vi "Acquire and process.vi"(7 "Rectangle":T2, 8 "error in (no error)":errorcluster, 9 "Substract images?":bool=TRUE, 10 "Image array":T1[](array[typedef]), 11 "Cam session":T3) -> (0 "error out":errorcluster, 2 "Trimmed image":T1, 3 "Mean Value":sgl)   [LabVIEW 2020]
doc: "Obtains the mean value a ROI maked by Rectangle. Is Substract images? is set toTrue, a difference is calculated between the base image and a newly acquired image before calculating the mean value."
uses:
  <vilib>/userdefined/High Color/IMAQdx.ctl
  <vilib>/vision/Image Controls.llb/IMAQ Image.ctl
  <vilib>/vision/driver/NI_Vision_Acquisition_Software.lvlib
  <vilib>/vision/NI_Vision_Development_Module.lvlib
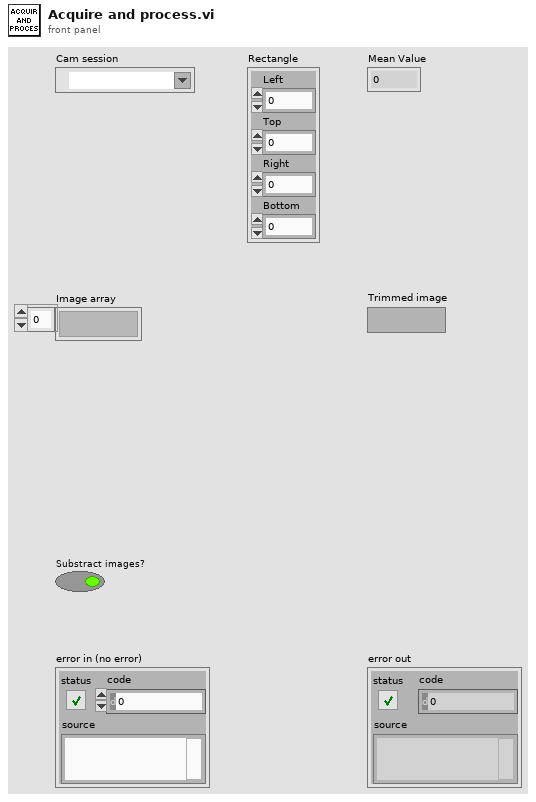
[diagram p1: front panel]
types:
  T1 = typedef "IMAQ Image.ctl" = refnum<image>
  T2 = cluster{"Left":i32, "Top":i32, "Right":i32, "Bottom":i32}
  T3 = typedef "IMAQdx.ctl" = refnum<k21>
  T4 = cluster{"Mean Value":sgl, "Standard Variation":sgl, "Minimal Value":sgl, "Maximal Value":sgl, "Area (calibrated)":sgl, "Area (pixels)":i32, "%":sgl}
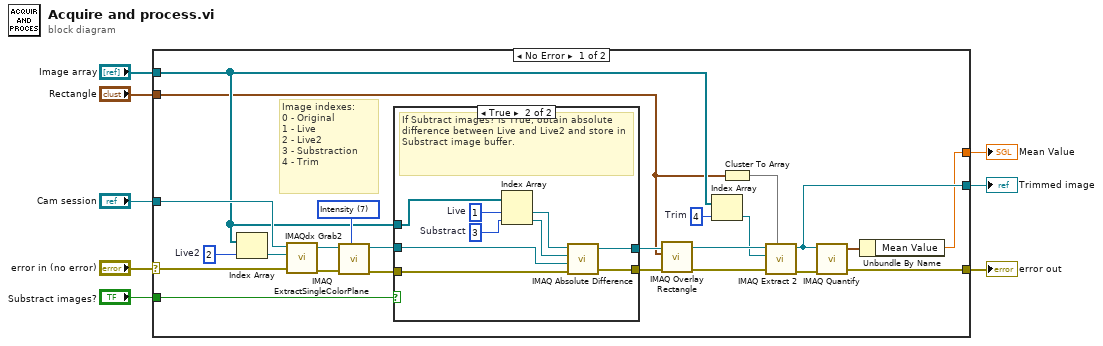
[diagram p0: block diagram]
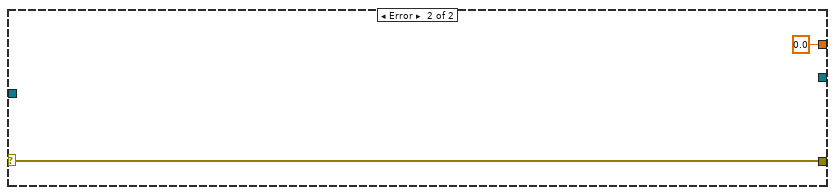
[diagram p3: hidden frame]
diagram:
  n1 = case shown="No Error" "error in (no error)" {
    selector: "error in (no error)" -> [w28 w45]
    tunnel: "Substract images?" -> [w32 _]
    tunnel: "Cam session" -> [w31 _]
    tunnel: "Image array" -> [w18 _]
    tunnel: "Rectangle" -> [w15 _]
    tunnel: [w12 _] -> w3
    tunnel: [w10 sgl 0.0 ("Mean Value")] -> w2
    tunnel: [w9 w45] -> w1
    frame No Error {
      w17 = 4  # Trim
      w29 = 2  # Live2
      w27 = 7 items=["Red", "Green", "Blue", "Hue", "Saturation", "Luminance", "Value", "Intensity"] ("Color Plane")
      # "Image indexes:\n0 - Original\n1 - Live\n2 - Live2\n3 - Substraction\n4 - Trim"
      n2 = Index Array(array=w18, index=w29) -> (element=w30:T1)
      n3 = call <vilib>:"IMAQdx Grab2.vi"("error in"=w28, "Image In"=w30, "Session In"=w31) -> ("error out"=w25:errorcluster, "Image Out"=w26:T1)  [unwired: 5 in, 2 out]
      n4 = call "IMAQ ExtractSingleColorPlane"("Color Plane"=w27, "error in (no error)"=w25, "Image Src"=w26) -> ("error out"=w24:errorcluster, "Image Dst Out"=w23:T1)  [unwired: 7 in]
      n5 = case shown="True" w32 {
        tunnel: w24 -> [w34 w43]
        tunnel: w18 -> [_ w42]
        tunnel: w23 -> [w33 w37]
        tunnel: [w34 w36] -> w22
        tunnel: [w33 w35] -> w21
        frame False {
          # "If Substract image? is False, pass image Live2 to be processed."
        }
        frame True {
          w38 = 3  # Substract
          w41 = 1  # Live
          # "If Subtract images? is True, obtain absolute difference between Live and Live2 and store in Substract image buffer."
          n6 = Index Array(array=w42, index #1=w41, index #2=w38) -> (element #1=w40:T1, element #2=w39:T1)
          n7 = call "IMAQ Absolute Difference"("Image Src A"=w40, "Image Dst"=w39, "Image Src B"=w37, "error in (no error)"=w43) -> ("Image Dst Out"=w35:T1, "error out"=w36:errorcluster)  [unwired: 3 in]
        }
      }
      n8 = call "IMAQ Overlay Rectangle"("error in (no error)"=w22, "Rectangle"=w15, "Image"=w21) -> ("error out"=w20:errorcluster, "Image Out"=w19:T1)  [unwired: 7 in]
      n9 = Index Array(array=w18, index=w17) -> (element=w16:T1)
      n10 = Cluster To Array(cluster=w15) -> (array=w14:i32[])
      n11 = call "IMAQ Extract 2"("Optional Rectangle"=w14, "error in (no error)"=w20, "Image Dst"=w16, "Image Src"=w19) -> ("error out"=w13:errorcluster, "Image Dst Out"=w12:T1)  [unwired: 6 in]
      n12 = call "IMAQ Quantify"("error in (no error)"=w13, "Image"=w12) -> ("error out"=w9:errorcluster, "Global Report"=w11:T4)  [unwired: 1 in, 1 out]
      n13 = Unbundle By Name(w11) -> ("Mean Value"=w10:sgl)
    }
    frame Error {
    }
  }
  "error out" <- w1
  "Mean Value" <- w2
  "Trimmed image" <- w3
